vi "Format Pipe String.vi"(8 "Grab samples":bool, 9 "Write File":bool, 11 "data":string) -> (0 "Samples":string, 1 "Key":string[](array[string]), 2 "Address C":string[](array[string]), 3 "Address U":string[](array[string]), 6 "path":path)   [LabVIEW 2020]
uses:
  <vilib>/Utility/file.llb/Write Delimited Spreadsheet (string).vi
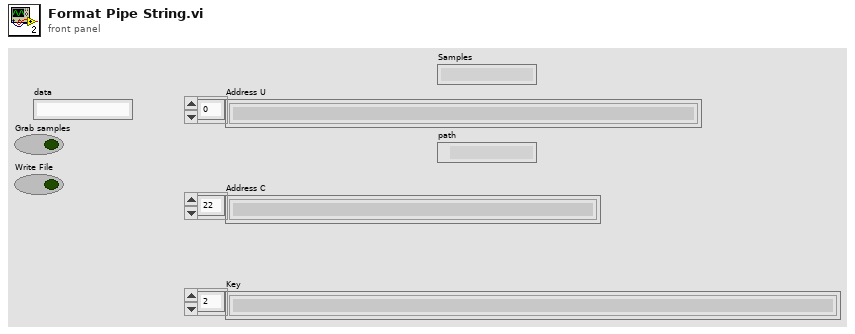
[diagram p1: front panel]
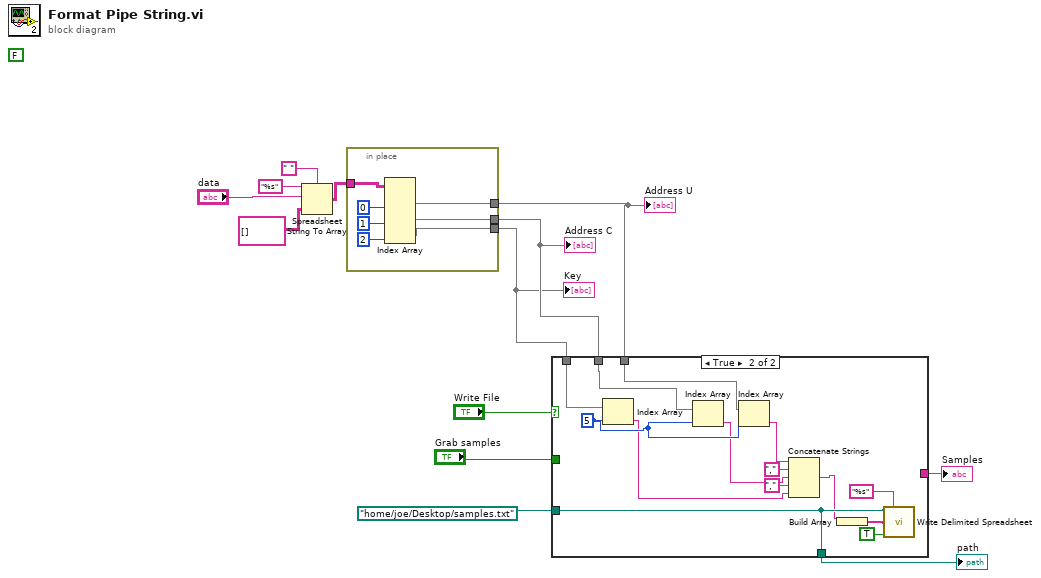
[diagram p0: block diagram]
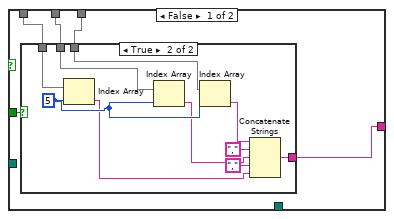
[diagram p2: hidden frame]
diagram:
  (unwired) FALSE
  n1 = Spreadsheet String To Array(delimiter (Tab)=" ", format string="%s", spreadsheet string="data", array type (2D Dbl)=string[][] [] ("appended array")) -> (array=w4:string[][])
  n2 = in-place {
    in-place-border: w4 -> [w20]
    in-place-border: [w19] -> w3
    in-place-border: [w18] -> w2
    in-place-border: [w14] -> w1
    n3 = Index Array(array=w20, index (col) #1=0 ("disabled index (col)"), index (col) #2=1 ("index (col)"), index (col) #3=2 ("index (col)")) -> (element #1=w19:string[], element #2=w18:string[], element #3=w14:string[])  [unwired: 3 in]
  }
  "Address U" <- w3
  "Address C" <- w2
  "Key" <- w1
  n4 = case shown="True" "Write File" {
    tunnel: w1 -> [w25 w49]
    tunnel: w2 -> [w24 w48]
    tunnel: w3 -> [w23 w47]
    tunnel: path "/home/joe/Desktop/samples.txt" ("path") -> [_ w37]
    tunnel: [_ w37] -> w8
    tunnel: [w22 _] -> w7
    tunnel: "Grab samples" -> [w21 _]
    frame False {
      n5 = case shown="True" w21 {
        tunnel: w25 -> [_ w29]
        tunnel: w24 -> [_ w28]
        tunnel: w23 -> [_ w27]
        tunnel: [_ w26] -> w22
        frame False {
        }
        frame True {
          w35 = 5 ("index")
          n6 = Index Array(array=w29, index=w35) -> (element=w30:string)
          n7 = Index Array(array=w28, index=w35) -> (element=w32:string)
          n8 = Index Array(array=w27, index=w35) -> (element=w34:string)
          n9 = Concatenate Strings(w34, "," ("string"), w32, "," ("string"), w30) -> (w26:string)
        }
      }
    }
    frame True {
      w46 = 5 ("index")
      n10 = Index Array(array=w49, index=w46) -> (element=w41:string)
      n11 = Index Array(array=w48, index=w46) -> (element=w43:string)
      n12 = Index Array(array=w47, index=w46) -> (element=w45:string)
      n13 = Concatenate Strings(w45, "," ("string"), w43, "," ("string"), w41) -> (w36:string)
      n14 = Build Array(w36) -> (w40:string[])
      n15 = call-poly <vilib>:"Write Delimited Spreadsheet.vi"("file path (dialog if empty)"=w37, "format (%s)"="%s", "1D data"=w40, "append to file? (new file:F)"=TRUE) -> ()  [unwired: 10 in, 2 out]
    }
  }
  "path" <- w8
  "Samples" <- w7
